vi "Sum.vi"(1 "Array":i32[](array[numeric])) -> (0 "Value":i32)   [LabVIEW 2018]
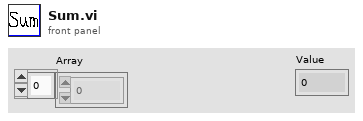
[diagram p1: front panel]
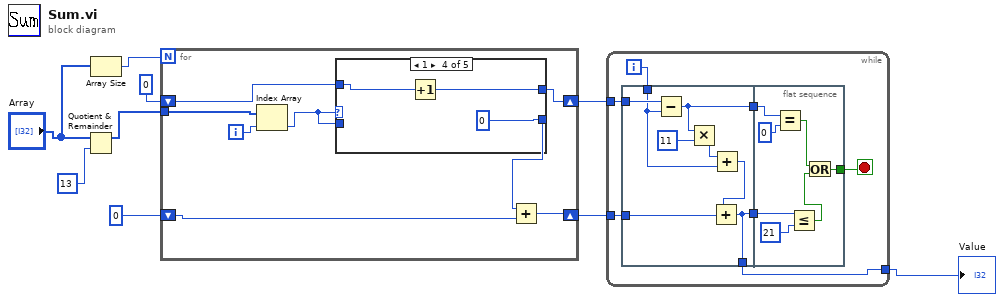
[diagram p0: block diagram]
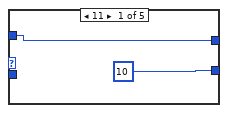
[diagram p2: hidden frame]
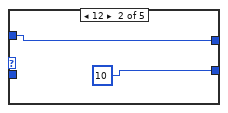
[diagram p3: hidden frame]
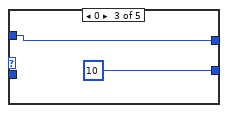
[diagram p4: hidden frame]
diagram:
  n1 = Quotient & Remainder(x="Array", y=13) -> (x-y*floor(x/y)=w5:i32[])  [unwired: 1 out]
  n2 = Array Size(array="Array") -> (size(s)=w7:i32)
  n3 = for {
    N: w7 -> [_]
    shift-right: [w12] -> w2
    shift-left: 0 -> [w17]
    tunnel: w5 -> [w16]
    shift-right: [w10] -> w3
    shift-left: 0 -> [w11]
    i -> [w15]
    n4 = Index Array(array=w16, index=w15) -> (element=w14:i32)
    n5 = case shown="1" w14 {
      tunnel: [10 10 10 0 w28] -> w13
      tunnel: w14 -> [_ _ _ _ w28]
      tunnel: w11 -> [w18 w20 w22 w25 w27]
      tunnel: [w18 w20 w22 w24 w27] -> w10
      frame 11 {
      }
      frame 12 {
      }
      frame 0 {
      }
      frame 1 {
        n6 = Increment(x=w25) -> (x+1=w24:i32)
      }
      frame 2, Default {
      }
    }
    n7 = Add(x=w13, y=w17) -> (x+y=w12:i32)
  }
  n8 = while {
    tunnel: w3 -> [w34]
    tunnel: w2 -> [w32]
    tunnel: [w30] -> w1
    i -> [w35]
    stop <- w29 stop-if-true
    n9 = flat-sequence {
      tunnel: w35 -> [w39]
      tunnel: w34 -> [w43]
      tunnel: [w41] -> w33
      tunnel: w32 -> [w38]
      tunnel: [w36] -> w31
      tunnel: [w36] -> w30
      tunnel: w33 -> [w50]
      tunnel: w31 -> [w48]
      tunnel: [w44] -> w29
      frame #0 {
        n10 = Subtract(x=w43, y=w39) -> (x-y=w41:i32)
        n11 = Multiply(x=w41, y=11) -> (x*y=w40:i32)
        n12 = Add(x=w40, y=w39) -> (x+y=w37:i32)
        n13 = Add(x=w37, y=w38) -> (x+y=w36:i32)
      }
      frame #1 {
        n14 = Equal?(x=w50, y=0) -> (x = y?=w46:bool)
        n15 = Less Or Equal?(x=w48, y=21) -> (x <= y?=w45:bool)
        n16 = Or(x=w46, y=w45) -> (x .or. y?=w44:bool)
      }
    }
  }
  "Value" <- w1
